vi "Joystick Input.vi"() -> ()   [LabVIEW 2025]
doc: "Joystick Input Example\n\nThis example takes input from a joystick (via the driver station) and displays it on the front panel.\n\nThis example expects a USB cable connected from your development PC to the Type B USB Jack (next to the power input) on the roboRIO.\n\nThis example requires the Driver Station to be running."
uses:
  <vilib>/Rock Robotics/WPI/Joystick/WPI_JoystickDeviceEnum.ctl
panel:
  out "X":dbl(slide) scale=-1.0..1.0
  out "Y":dbl(slide) scale=1.0..-1.0
  out "XY Graph":cluster{dbl, dbl}[](graph)
  in  "Joystick Port":T1
  in  "stop":bool
  # "This example requires the Driver Station to be running."
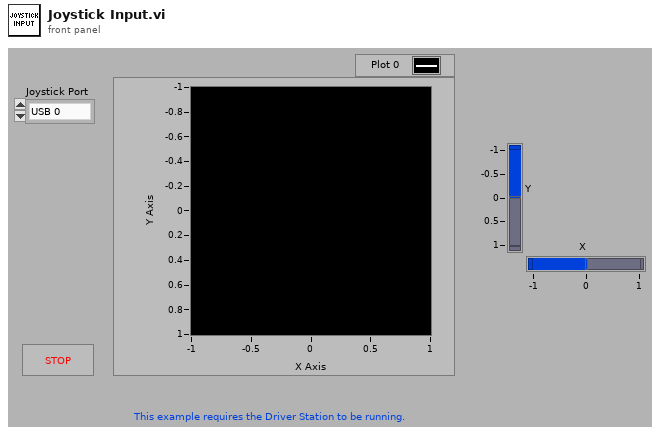
[diagram p1: front panel]
types:
  T1 = typedef "WPI_JoystickDeviceEnum.ctl" = enum16{"USB 0", "USB 1", "USB 2", "USB 3", "USB 4", "USB 5"}
  T2 = typedef "WPI_JoystickDevRef.ctl" = cluster{"Device":T1}
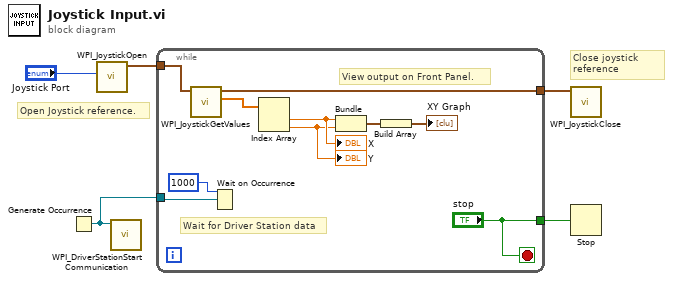
[diagram p0: block diagram]
diagram:
  # "Close joystick reference"
  # "Open Joystick reference."
  n1 = Generate Occurrence() -> (w3:refnum<k4>)
  n2 = call <vilib>:"WPI_JoystickOpen.vi"("JoystickDevice"="Joystick Port") -> ("JoystickDevRef"=w5:T2)  [unwired: 10 out]
  n3 = call <vilib>:"WPI_DriverStationStart Communication.vi"("occurrence"=w3) -> ()  [unwired: 2 in, 9 out]
  n4 = while {
    tunnel: w5 -> [w13]
    tunnel: ["stop"] -> w1
    tunnel: w3 -> [w14]
    tunnel: [w12] -> w2
    stop <- "stop" stop-if-true
    # "Wait for Driver Station data"
    # "View output on Front Panel."
    n5 = call <vilib>:"WPI_JoystickGetValues.vi"("JoystickDevRef"=w13) -> ("Axes"=w11:dbl[], "JoystickDevRef"=w12:T2)  [unwired: 6 in, 3 out]
    n6 = Wait on Occurrence(2:w14, 3:1000 ("ms timeout (-1)")) -> ()  [unwired: 2 out]
    n7 = Index Array(array=w11) -> (element #1=w8:dbl, element #2=w6:dbl)  [unwired: 2 in]
    "Y" <- w6
    "X" <- w8
    n8 = Bundle("upper limit"=w8, "upper limit"=w6) -> (w10:cluster{"upper limit":dbl, "upper limit":dbl})  [unwired: 1 out]
    n9 = Build Array(w10) -> (→"XY Graph":cluster{"upper limit":dbl, "upper limit":dbl}[])
  }
  n10 = call <vilib>:"WPI_JoystickClose.vi"("JoystickDevRef"=w2) -> ()  [unwired: 11 out]
  n11 = Stop(stop? (T)=w1) -> ()
